vi "Open Device.vi"(8 "error in":errorcluster, 11 "Port":string) -> (0 "error out":errorcluster, 3 ".NET Refnum out":refnum<k24>)   [LabVIEW 2019, in "ESP301-Driver.lvlib"]
uses:
  ESP301-Driver.lvlib
  Newport.ESP301.CommandInterface
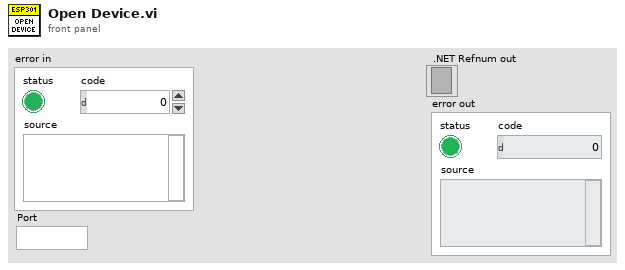
[diagram p1: front panel]
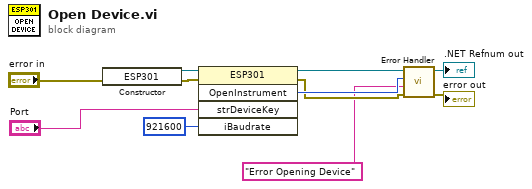
[diagram p0: block diagram]
diagram:
  n1 = constructor class="ESP301"(error in="error in") -> (reference out=w10:refnum<k24>, error out=w11:errorcluster)  [unwired: 2 in, 1 out]
  n2 = invoke class="ESP301" method="OpenInstrument"(reference=w10, error in=w11, "strDeviceKey"="Port", "iBaudrate"=921600) -> (reference out=w6:refnum<k24>, error out=w4:errorcluster, "OpenInstrument"=w5:i32)  [unwired: 1 in, 2 out]
  n3 = call "Error Handler.vi"("error in (no error)"=w4, "Message"="Error Opening Device", "Error Code"=w5, ".NET Refnum in"=w6) -> ("error out"=→"error out":errorcluster, ".NET Refnum out"=→".NET Refnum out":refnum<k24>)  [unwired: 6 in]
